vi "S7_Read.vi"(0 "TCP":refnum<k5>, 1 "DB #":u16=1, 2 "读取长度":u16=1, 5 "寄存器类型":u8(ring)=128 items=["I/O (P)"=128, "Input (I)"=129, "Output (Q)"=130, "Bit Memory (M)"=131, "Data (DB)"=132, "Instance Data (DI)"=133, "Local Data (L)"=134, "Predecessor Local Data (VL)"=135], 7 "起始地址":u32=131, 9 "数据类型":u16(ring) items=["byte", "word", "Dword"], 11 "error in":errorcluster) -> (4 "TCP":refnum<k5>, 6 "数据":u32[](array[numeric]), 8 "读取成功":bool, 15 "error out":errorcluster)   [LabVIEW 2018]
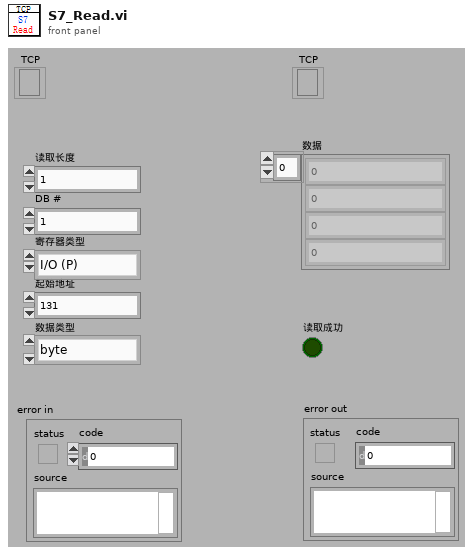
[diagram p1: front panel]
types:
  T1 = enum16{"Standard", "Buffered", "CRLF", "Immediate"}
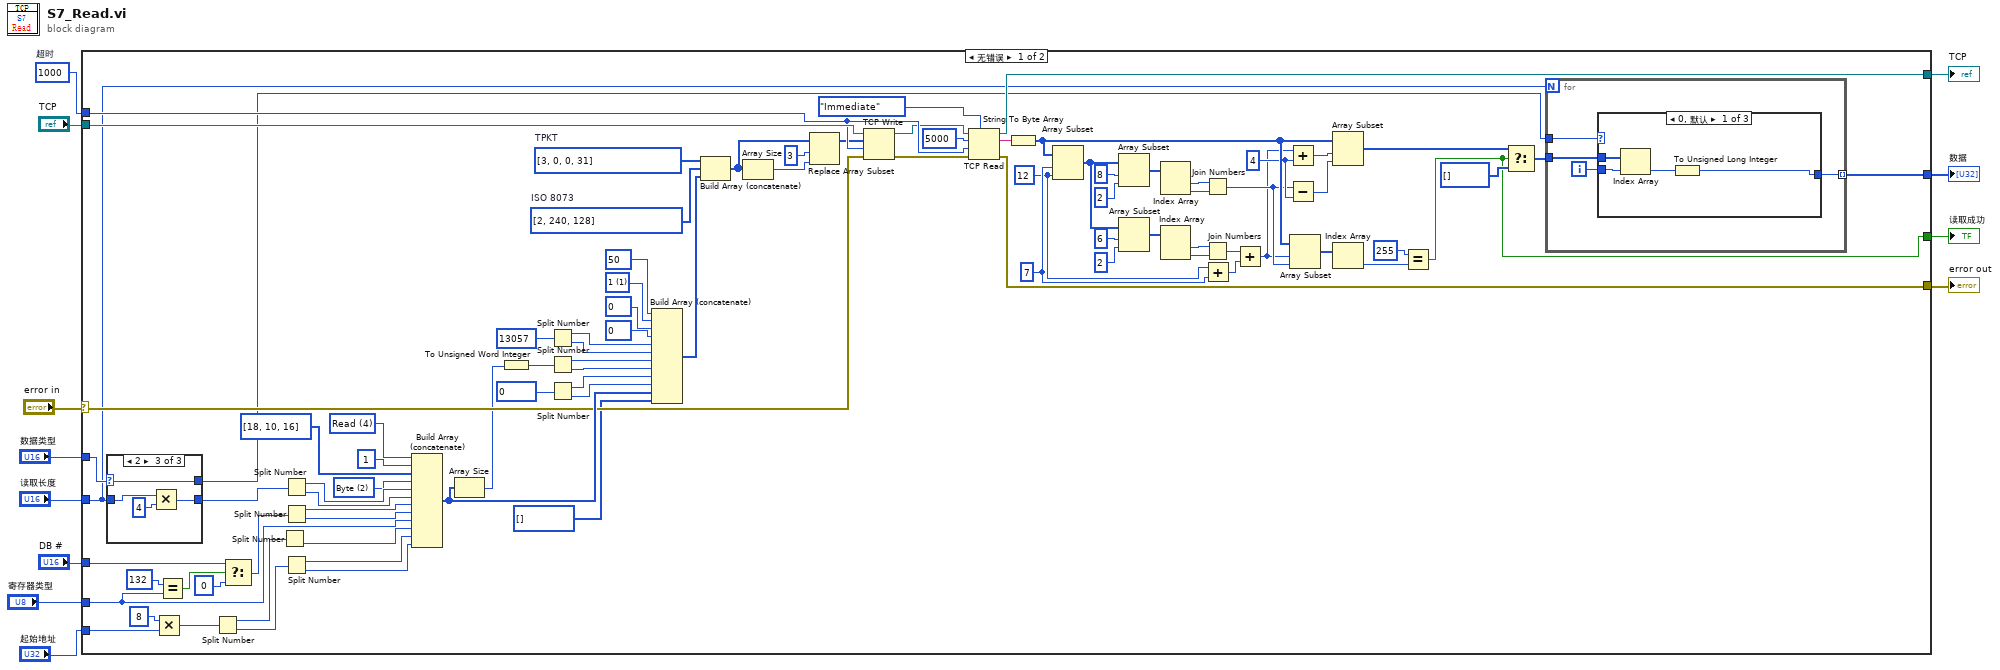
[diagram p0: block diagram]
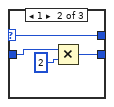
[diagram p3: hidden frame]
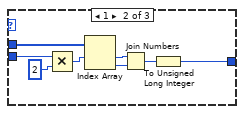
[diagram p4: hidden frame]
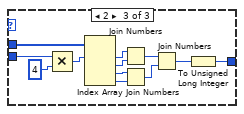
[diagram p5: hidden frame]
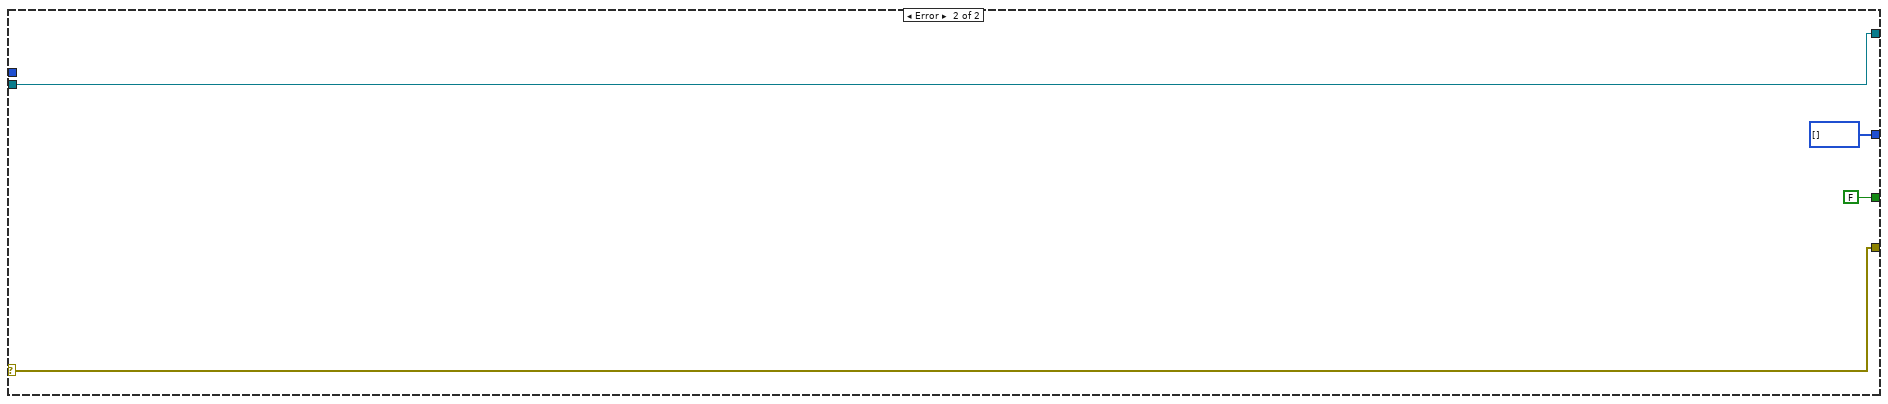
[diagram p6: hidden frame]
diagram:
  w10 = u32 1000  # 超时
  n1 = case shown="无错误" "error in" {
    selector: "error in" -> [w81 w141]
    tunnel: "TCP" -> [w100 w142]
    tunnel: w10 -> [w98 _]
    tunnel: "读取长度" -> [w13 _]
    tunnel: "DB #" -> [w86 _]
    tunnel: "起始地址" -> [w84 _]
    tunnel: "寄存器类型" -> [w85 _]
    tunnel: [w99 w142] -> w11
    tunnel: [w77 w141] -> w9
    tunnel: [w97 u8[] [] ("f")] -> w8
    tunnel: [w79 FALSE ("Data Valid")] -> w7
    tunnel: "数据类型" -> [w16 _]
    frame No Error {
      w54 = u8 1 items=["1"=1, "2"=2, "3"=3, "7"=7]
      w58 = u8 4 items=["Read"=4, "Write"=5] ("Read / Write")
      w63 = u8 2 items=["Bit"=1, "Byte"=2, "Word"=4, "Dword"=6] ("Transport Type")
      w40 = u8[] [3, 0, 0, 31]  # TPKT
      w39 = 4 ("y")
      w18 = 12 ("length")
      w19 = 7 ("index")
      w42 = u8[] [2, 240, 128]  # ISO 8073
      n2 = case shown="2" w16 {
        selector: w16 -> [w101 w103 w107]
        tunnel: w13 -> [w102 w105 w110]
        tunnel: [w102 w104 w108] -> w15
        tunnel: [w101 w103 w107] -> w14
        frame 0, Default {
        }
        frame 1 {
          n3 = Multiply(x=w105, y=u16 2) -> (x*y=w104:u16)
        }
        frame 2 {
          n4 = Multiply(x=w110, y=u16 4) -> (x*y=w108:u16)
        }
      }
      n5 = Multiply(x=u32 8 ("y"), y=w84) -> (x*y=w61:u32)
      n6 = Equal?(x=u8 132, y=w85) -> (x = y?=w69:bool)
      n7 = Split Number(x=w61) -> (hi(x)=w76:u16, lo(x)=w75:u16)
      n8 = Select(t=w86, s=w69, f=u16 0 ("Sequence #")) -> (s? t:f=w64:u16)
      n9 = Split Number(x=w76) -> (lo(x)=w72:u8)  [unwired: 1 out]
      n10 = Split Number(x=w15) -> (hi(x)=w73:u8, lo(x)=w62:u8)
      n11 = Split Number(x=w64) -> (hi(x)=w65:u8, lo(x)=w66:u8)
      n12 = Split Number(x=w75) -> (hi(x)=w71:u8, lo(x)=w70:u8)
      n13 = Build Array (concatenate)(w58, u8 1 ("Sequence #"), u8[] [18, 10, 16] ("Msg Header"), w63, w73, w62, w65, w66, w85, w72, w71, w70) -> (w83:u8[])
      n14 = Array Size(array=w83) -> (size(s)=w45:i32)
      n15 = To Unsigned Word Integer(number=w45) -> (unsigned 16bit integer=w44:u16)
      n16 = Split Number(x=u16 13057 ("DLE")) -> (hi(x)=w47:u8, lo(x)=w46:u8)
      n17 = Split Number(x=w44) -> (hi(x)=w57:u8, lo(x)=w52:u8)
      n18 = Split Number(x=u16 0 ("DLE")) -> (hi(x)=w51:u8, lo(x)=w50:u8)
      n19 = Build Array (concatenate)(u8 50 ("DLE"), w54, u8 0 ("DLE"), u8 0 ("DLE"), w47, w46, w57, w52, w51, w50, w83, u8[] []) -> (w41:u8[])
      n20 = Build Array (concatenate)(w40, w42, w41) -> (w82:u8[])
      n21 = Array Size(array=w82) -> (size(s)=w87:i32)
      n22 = Replace Array Subset(array=w82, new element=w87, index=3) -> (w89:u8[])
      n23 = TCP Write(connection ID=w100, data in=w89, error in (no error)=w81, 9:w98) -> (connection ID out=w94:refnum<k5>, error out=w93:errorcluster)  [unwired: 1 out]
      n24 = TCP Read(connection ID=w94, bytes to read=5000, error in (no error)=w93, 7:T1."Immediate" ("mode (standard)"), 9:w98) -> (connection ID out=w99:refnum<k5>, data out=w92:string, error out=w77:errorcluster)
      n25 = String To Byte Array(string=w92) -> (unsigned byte array=w80:u8[])
      n26 = Array Subset(array=w80, index=w19, length=w18) -> (w24:u8[])
      n27 = Array Subset(array=w24, index=8, length=2) -> (w30:u8[])
      n28 = Array Subset(array=w24, index=6, length=2) -> (w25:u8[])
      n29 = Index Array(array=w30) -> (element #1=w29:u8, element #2=w28:u8)  [unwired: 2 in]
      n30 = Index Array(array=w25) -> (element #1=w26:u8, element #2=w27:u8)  [unwired: 2 in]
      n31 = Join Numbers(hi=w29, lo=w28) -> ((hi.lo)=w38:u16)
      n32 = Join Numbers(hi=w26, lo=w27) -> ((hi.lo)=w31:u16)
      n33 = Add(x=w18, y=w19) -> (x+y=w17:i32)
      n34 = Add(x=w31, y=w17) -> (x+y=w34:i32)
      n35 = Add(x=w34, y=w39) -> (x+y=w36:i32)
      n36 = Subtract(x=w38, y=w39) -> (x-y=w37:i32)
      n37 = Array Subset(array=w80, index=w34, length=w38) -> (w35:u8[])
      n38 = Array Subset(array=w80, index=w36, length=w37) -> (w78:u8[])
      n39 = Index Array(array=w35) -> (element=w33:u8)  [unwired: 1 in]
      n40 = Equal?(x=u8 255, y=w33) -> (x = y?=w79:bool)
      n41 = Select(t=w78, s=w79, f=u8[] []) -> (s? t:f=w96:u8[])
      n42 = for {
        N: w13 -> [_]
        tunnel: w96 -> [w113]
        tunnel: w14 -> [w112]
        tunnel: [w114] -> w97 mode=indexing
        i -> [w111]
        n43 = case shown="0, 默认" w112 {
          tunnel: [w118 w126 w131] -> w114
          tunnel: w113 -> [w116 w122 w130]
          tunnel: w111 -> [w115 w121 w129]
          frame 0, Default {
            n44 = Index Array(array=w116, index=w115) -> (element=w117:u8)
            n45 = To Unsigned Long Integer(number=w117) -> (unsigned 32bit integer=w118:u32)
          }
          frame 1 {
            n46 = Multiply(x=w121, y=2) -> (x*y=w119:i32)
            n47 = Index Array(array=w122, index #1=w119) -> (element #1=w125:u8, element #2=w124:u8)  [unwired: 1 in]
            n48 = Join Numbers(hi=w125, lo=w124) -> ((hi.lo)=w123:u16)
            n49 = To Unsigned Long Integer(number=w123) -> (unsigned 32bit integer=w126:u32)
          }
          frame 2 {
            n50 = Multiply(x=w129, y=4) -> (x*y=w127:i32)
            n51 = Index Array(array=w130, index #1=w127) -> (element #1=w138:u8, element #2=w137:u8, element #3=w136:u8, element #4=w135:u8)  [unwired: 3 in]
            n52 = Join Numbers(hi=w138, lo=w137) -> ((hi.lo)=w134:u16)
            n53 = Join Numbers(hi=w136, lo=w135) -> ((hi.lo)=w133:u16)
            n54 = Join Numbers(hi=w134, lo=w133) -> ((hi.lo)=w132:u32)
            n55 = To Unsigned Long Integer(number=w132) -> (unsigned 32bit integer=w131:u32)
          }
        }
      }
    }
    frame Error {
    }
  }
  "TCP" <- w11
  "error out" <- w9
  "数据" <- w8
  "读取成功" <- w7
